vi "Query.vi"(7 "LabVIEW Web Service Request":refnum<class "Web Request.lvclass">) -> ()   [LabVIEW 2016]
uses:
  <vilib>/wsapi/Web Request.lvclass
  Device Info.ctl
  Inventory FGV Command.ctl
  <vilib>/NI_Real-Time Target Support.lvlib
panel:
  out "error out":errorcluster
  # "Use the Web Service Request input terminal to call the VIs on the Web Services palette. Do not remove it from the connector pane unless you don't need access to the palette."
  # "Each additional control wired to the connector pane will be available as an input in the URL. To include an indicator in terminal-mode output (the default setting), it must also be wired to the connector pane."
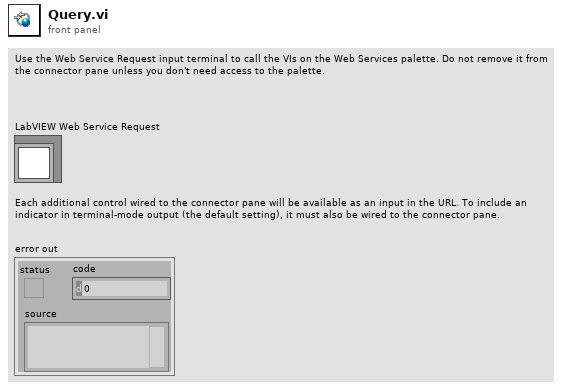
[diagram p1: front panel]
types:
  T1 = typedef "Inventory FGV Command.ctl" = enum16{"Load Items", "Check Status", "Return Items", "Check Out Items", "Add New Item", "Get All Items", "Remove Item", "Search"}
  T2 = typedef "Device Info.ctl" = cluster{"Model Number":string, "Identifier":string, "Available?":bool, "Owner":string, "Owner Email":string, "Last Activity Date":string, "Loan Purpose":string, "Department":string, "Notes":string, "Serial Number":string}
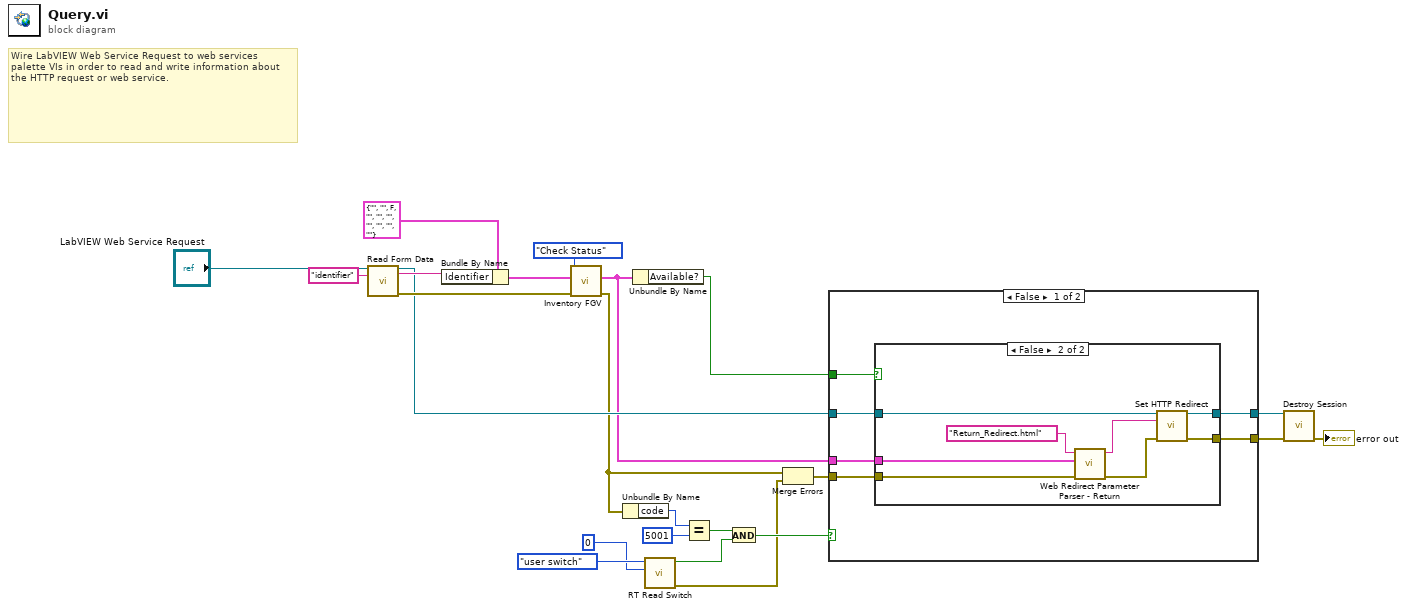
[diagram p0: block diagram]
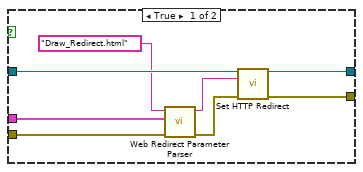
[diagram p2: hidden frame]
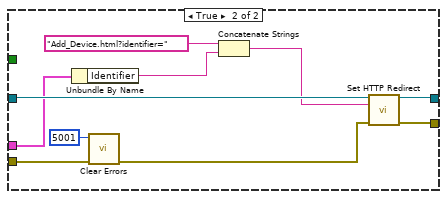
[diagram p3: hidden frame]
diagram:
  # "Wire LabVIEW Web Service Request to web services palette VIs in order to read and write information about the HTTP request or web service."
  n1 = call <vilib>:"Read Form Data.vi"("LabVIEW Web Service Request"="LabVIEW Web Service Request", "key"="identifier") -> ("LabVIEW Web Service Request out"=w18:refnum<class "Web Request.lvclass">, "value"=w20:string, "error out"=w19:errorcluster)  [unwired: 10 in, 1 out]
  n2 = Bundle By Name(cluster=T2 {"Model Number"="", "Identifier"="", "Available?"=FALSE, "Owner"="", "Owner Email"="", "Last Activity Date"="", "Loan Purpose"="", "Department"="", "Notes"="", "Serial Number"=""} ("Device"), "Identifier"=w20) -> (w17:T2)
  n3 = call "Inventory FGV.vi"("error in"=w19, "Device Info"=w17, "Command"=Inventory_FGV_Command."Check Status") -> ("error out"=w2:errorcluster, "Device Info Out"=w12:T2)  [unwired: 5 in, 1 out]
  n4 = Unbundle By Name(w2) -> ("code"=w8:i32)
  n5 = Unbundle By Name(w12) -> ("Available?"=w16:bool)
  n6 = call <vilib>:"RT Read Switch.vi"("switch ID"=0, "switch type (system switch)"=enum16{"system switch", "user switch"}."user switch") -> ("error out"=w1:errorcluster, "switch state (on/off)"=w5:bool)  [unwired: 8 in]
  n7 = Equal?(x=w8, y=5001) -> (x = y?=w6:bool)
  n8 = And(x=w6, y=w5) -> (x .and. y?=w4:bool)
  n9 = Merge Errors(w2, w1) -> (w3:errorcluster)
  n10 = case shown="False" w4 {
    tunnel: w18 -> [w29 w50]
    tunnel: w16 -> [w28 _]
    tunnel: [w27 w51] -> w15
    tunnel: [w26 w52] -> w14
    tunnel: w12 -> [w25 w49]
    tunnel: w3 -> [w24 w55]
    frame False {
      n11 = case shown="False" w28 {
        tunnel: w29 -> [w37 w45]
        tunnel: w24 -> [w30 w42]
        tunnel: [w36 w44] -> w26
        tunnel: w25 -> [w31 w41]
        tunnel: [w35 w43] -> w27
        frame True {
          n12 = call "Web Redirect Parameter Parser.vi"("redirect URL"="Draw_Redirect.html", "Device"=w31, "error in (no error)"=w30) -> ("Output String"=w33:string, "error out"=w32:errorcluster)  [unwired: 6 in]
          n13 = call <vilib>:"Set HTTP Redirect.vi"("LabVIEW Web Service Request"=w37, "redirect URL"=w33, "error in (no error)"=w32) -> ("LabVIEW Web Service Request out"=w35:refnum<class "Web Request.lvclass">, "error out"=w36:errorcluster)  [unwired: 11 in]
        }
        frame False {
          n14 = call "Web Redirect Parameter Parser - Return.vi"("redirect URL"="Return_Redirect.html", "Device"=w41, "error in (no error)"=w42) -> ("Output String"=w38:string, "error out"=w39:errorcluster)  [unwired: 6 in]
          n15 = call <vilib>:"Set HTTP Redirect.vi"("LabVIEW Web Service Request"=w45, "redirect URL"=w38, "error in (no error)"=w39) -> ("LabVIEW Web Service Request out"=w43:refnum<class "Web Request.lvclass">, "error out"=w44:errorcluster)  [unwired: 11 in]
        }
      }
    }
    frame True {
      n16 = Unbundle By Name(w49) -> ("Identifier"=w47:string)
      n17 = call <vilib>:"Clear Errors.vi"("error in (no error)"=w55, "specific error code to clear (0: all)"=5001) -> ("error out"=w53:errorcluster)  [unwired: 4 in, 1 out]
      n18 = Concatenate Strings("Add_Device.html?identifier=", w47) -> (w46:string)
      n19 = call <vilib>:"Set HTTP Redirect.vi"("LabVIEW Web Service Request"=w50, "redirect URL"=w46, "error in (no error)"=w53) -> ("LabVIEW Web Service Request out"=w51:refnum<class "Web Request.lvclass">, "error out"=w52:errorcluster)  [unwired: 11 in]
    }
  }
  n20 = call <vilib>:"Destroy Session.vi"("LabVIEW Web Service Request"=w15, "error in (no error)"=w14) -> ("error out"=→"error out":errorcluster)  [unwired: 12 in, 1 out]
